vi "Boolean Assert Test.vi"(11 "Data In":bool) -> (3 "Data Out":bool)   [LabVIEW 2018]
uses:
  Core/Assert API Components/Failure Actions.ctl
  Core/Assert API Components/Assert API Components.lvlib
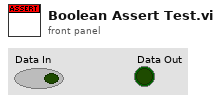
[diagram p1: front panel]
types:
  T1 = typedef "Assert API Components.lvlib/Failure Actions.ctl" = enum16{"None", "Log To File", "Pause Execution", "Abort Execution"}
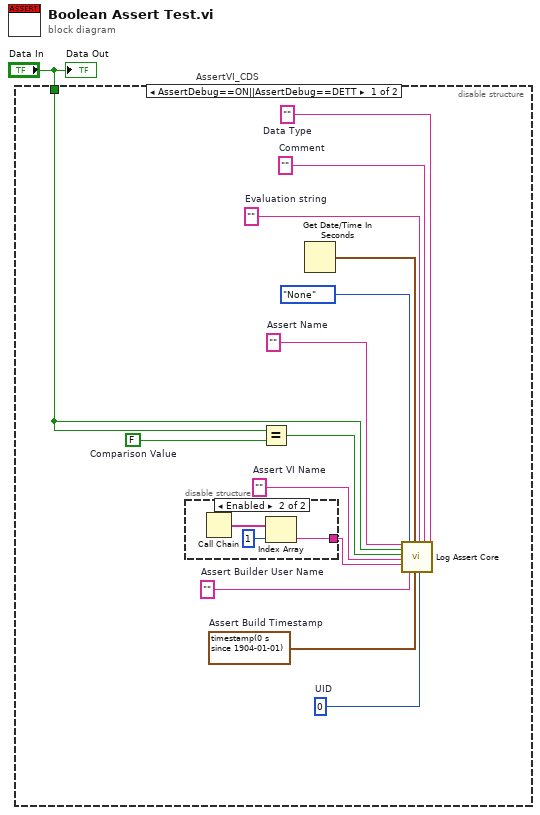
[diagram p0: block diagram]
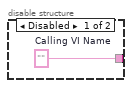
[diagram p2: hidden frame]
diagram:
  n1 = disable-structure "AssertVI_CDS" shown="AssertDebug==ON||AssertDebug==DETT" {
    disable-tunnel: "Data In" -> [w12 _]
    frame condition #0 (active) {
      w2 = 0  # UID
      w5 = ""  # Assert VI Name
      w7 = timestamp(0 s since 1904-01-01)  # Assert Build Timestamp
      w8 = ""  # Assert Builder User Name
      w9 = ""  # Data Type
      w14 = ""  # Comment
      w13 = ""  # Evaluation string
      w15 = ""  # Assert Name
      w11 = FALSE  # Comparison Value
      n2 = disable-structure shown="Enabled" {
        disable-tunnel: [w16 w17] -> w6
        frame Disabled {
          w16 = ""  # Calling VI Name
        }
        frame Enabled {
          n3 = Call Chain() -> (call chain=w18:string[])
          n4 = Index Array(array=w18, index=1) -> (element=w17:string)
        }
      }
      n5 = Equal?(x=w12, y=w11) -> (x = y?=w10:bool)
      n6 = Get Date/Time In Seconds() -> (seconds since 1Jan1904=w3:timestamp)
      n7 = call "Log Assert Core.vi"("Assert Name"=w15, "Data Value"=w12, "Status"=w10, "Assert VI Name"=w5, "Calling VI Name"=w6, "Failure Action"=Failure_Actions."None" ("Default Failure Action"), "Assert Builder User Name"=w8, "Last Update"=w3, "Assert Build Timestamp"=w7, "Evaluation String"=w13, "Assert VI UID"=w2, "Comment"=w14, "Data Type"=w9) -> ()  [unwired: 7 in]
    }
    frame condition #1 {
    }
  }
  "Data Out" <- "Data In"
